vi "IMAQ FPGA Camera Link Data to Pixels 4 Tap 10-Bit.vi"(1 "Camera Link Data":T1) -> (0 "Pixels":u16[](array[numeric]))   [LabVIEW 2017]
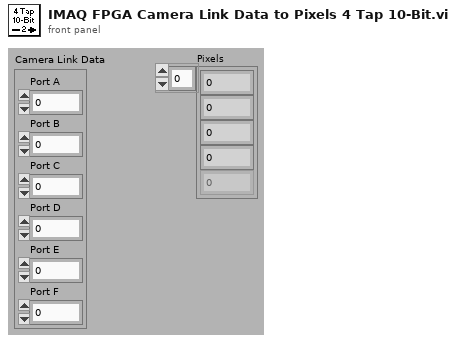
[diagram p1: front panel]
types:
  T1 = cluster{"Port A":u8, "Port B":u8, "Port C":u8, "Port D":u8, "Port E":u8, "Port F":u8}
  T2 = cluster{"Pixel 0":u16, "Pixel 1":u16, "Pixel 2":u16, "Pixel 3":u16}
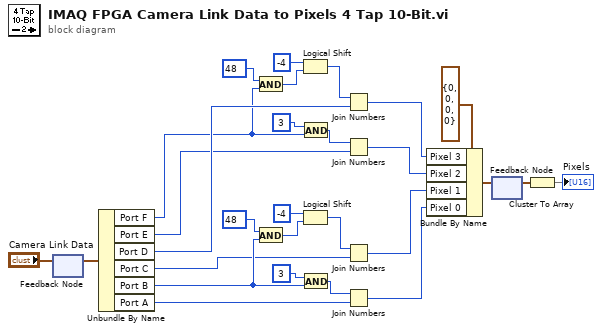
[diagram p0: block diagram]
diagram:
  n1 = feedback-in #1("Camera Link Data") -> ()
  n2 = feedback #1() -> (w3:T1)  [unwired: 1 in]
  n3 = Unbundle By Name(w3) -> ("Port F"=w5:u8, "Port E"=w6:u8, "Port D"=w7:u8, "Port C"=w8:u8, "Port B"=w9:u8, "Port A"=w10:u8)
  n4 = And(x=u8 48 ("hi"), y=w5) -> (x .and. y?=w17:u8)
  n5 = And(x=u8 48 ("hi"), y=w9) -> (x .and. y?=w25:u8)
  n6 = Logical Shift(y=i8 -4, x=w17) -> (x << y=w19:u8)
  n7 = Logical Shift(y=i8 -4, x=w25) -> (x << y=w23:u8)
  n8 = And(x=u8 3 ("hi"), y=w5) -> (x .and. y?=w15:u8)
  n9 = And(x=u8 3 ("hi"), y=w9) -> (x .and. y?=w27:u8)
  n10 = Join Numbers(hi=w19, lo=w7) -> ((hi.lo)=w13:u16)
  n11 = Join Numbers(hi=w15, lo=w6) -> ((hi.lo)=w12:u16)
  n12 = Join Numbers(hi=w23, lo=w8) -> ((hi.lo)=w21:u16)
  n13 = Join Numbers(hi=w27, lo=w10) -> ((hi.lo)=w22:u16)
  n14 = Bundle By Name(cluster=T2 {"Pixel 0"=0, "Pixel 1"=0, "Pixel 2"=0, "Pixel 3"=0} ("PixelData"), "Pixel 3"=w13, "Pixel 2"=w12, "Pixel 1"=w21, "Pixel 0"=w22) -> (w2:T2)
  n15 = feedback #2() -> (w1:T2)  [unwired: 1 in]
  n16 = feedback-in #2(w2) -> ()
  n17 = Cluster To Array(cluster=w1) -> (array=→"Pixels":u16[])
